vi "VI_Principal.vi"() -> ()   [LabVIEW 2024]
uses:
  <vilib>/LabVIEW Open Source Project/Epoch Date & Time/epoch.UNIX/Epoch.UNIX.lvclass
panel:
  in  "Tab Control":enum32{"Page 1", "Page 2", "Page 3"}(tab)
  out "POTENCIA  A":waveform(dbl)(graph)
  out "FASE B":waveform(dbl)
  out "POTENCIA   B":waveform(dbl)(graph)
  out "output waveform":waveform(dbl)
  out "POTENCIA CC":waveform(dbl)(graph)
  out "FASE C":dbl(graph)
  out "FASE A":waveform(dbl)(graph)
  in  "stop 2":bool
  out "Waveform Chart 3":waveform(dbl)(graph)
  in  "stop":bool
  out "Waveform Chart 2":waveform(dbl)(graph)
  out "Waveform Chart":dbl(graph)
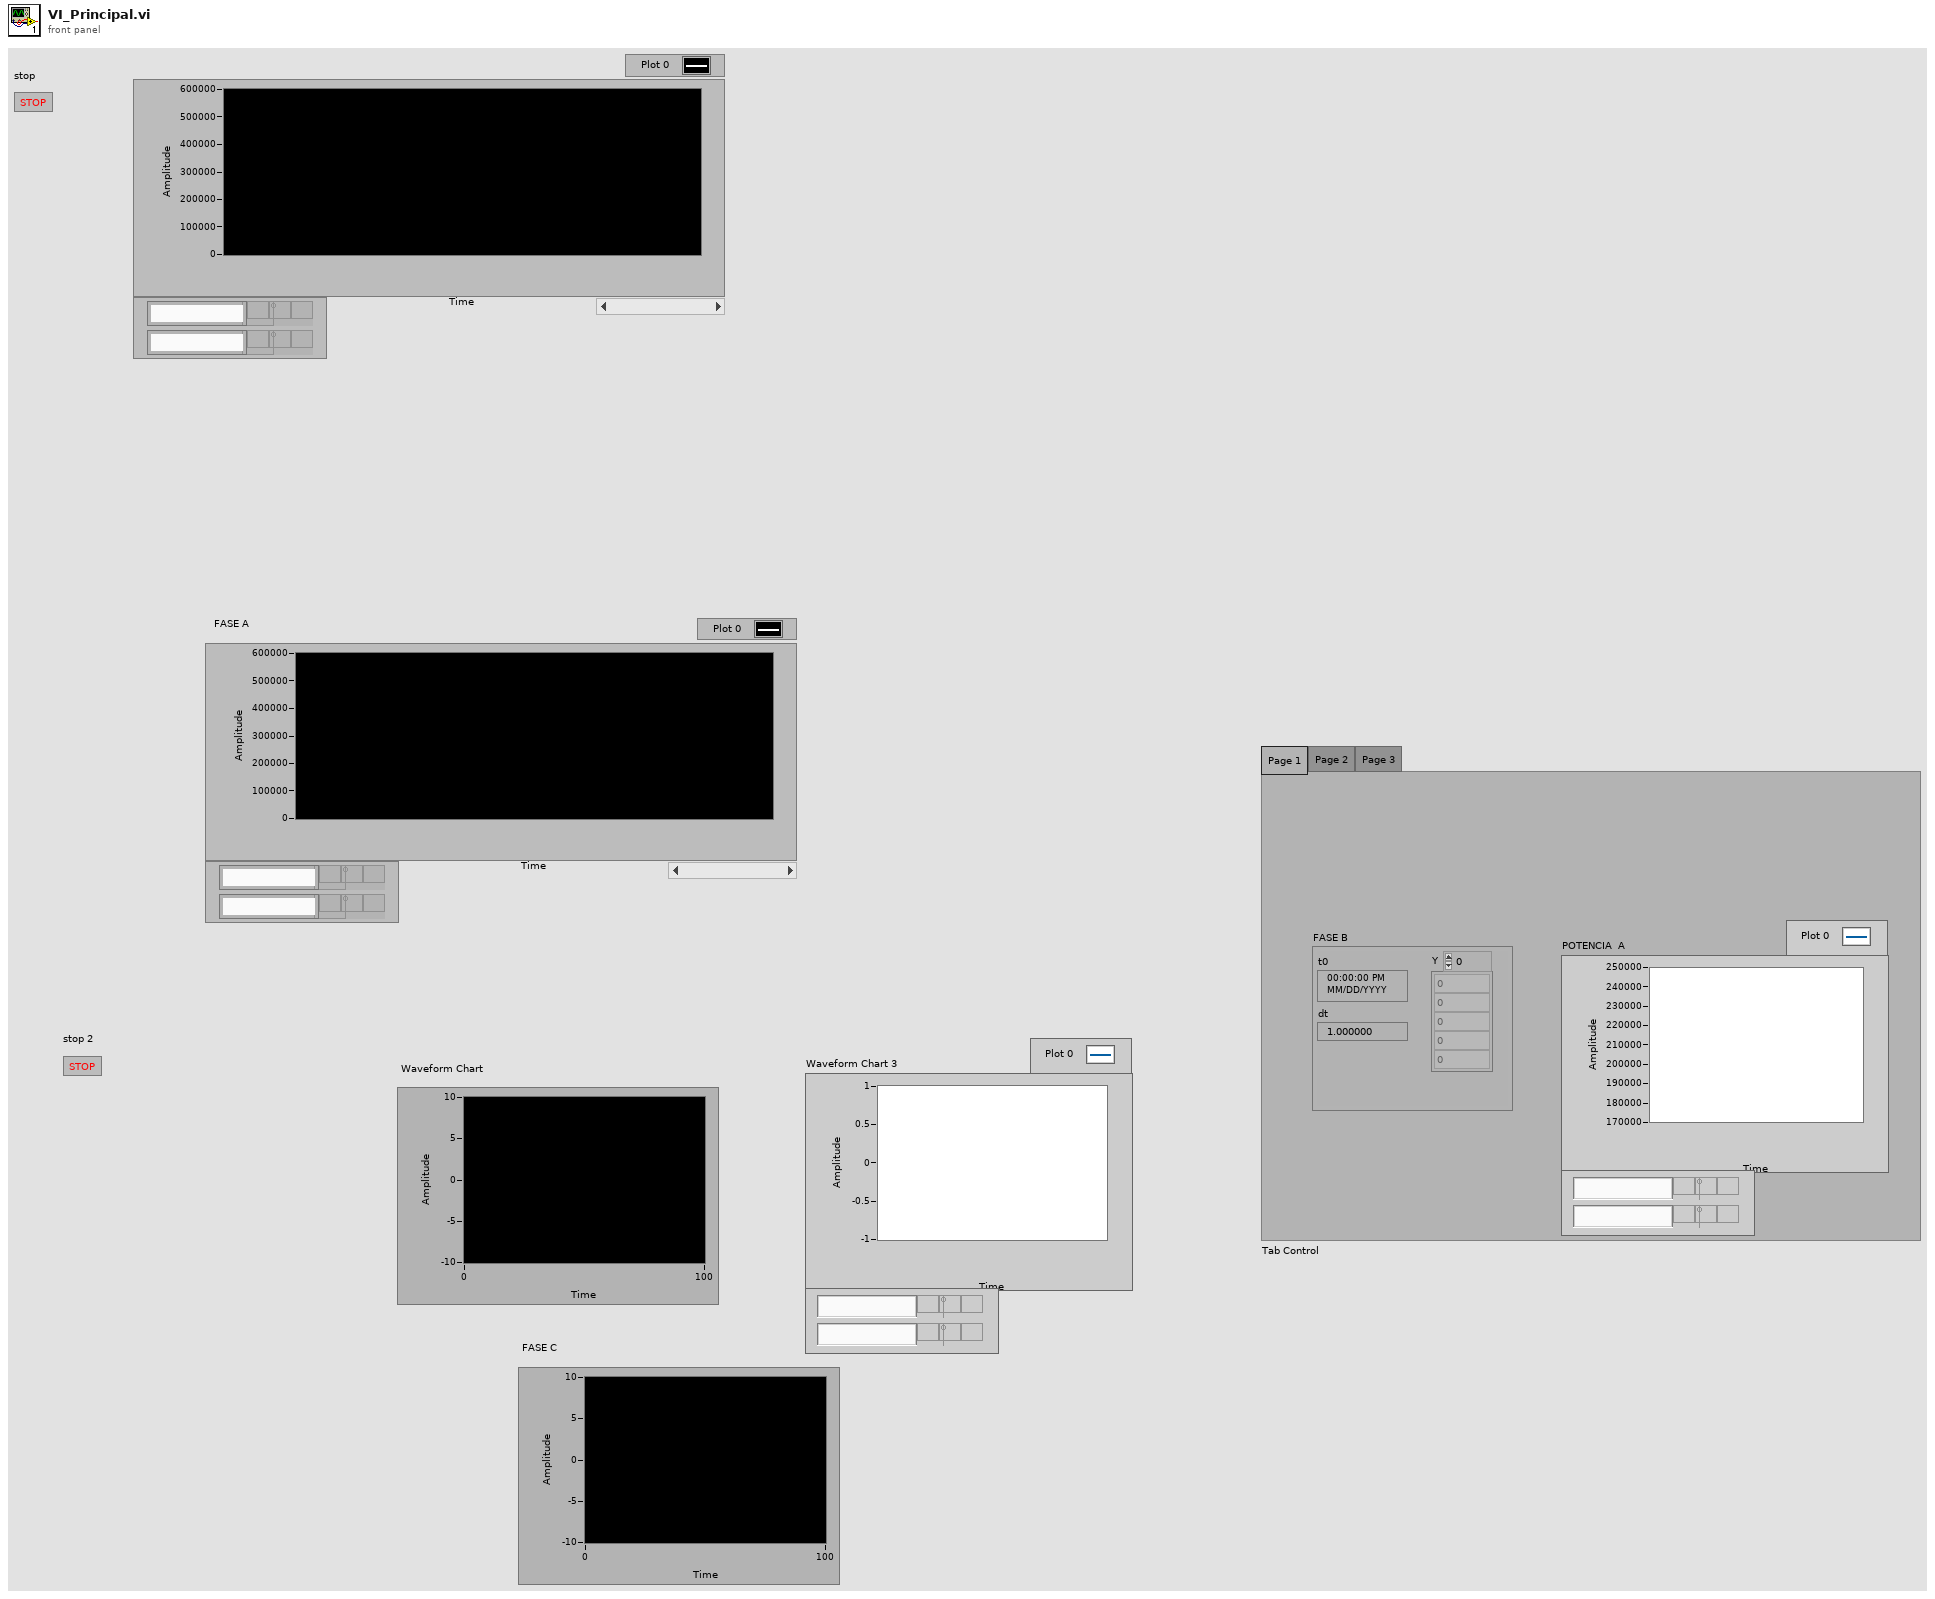
[diagram p1: front panel]
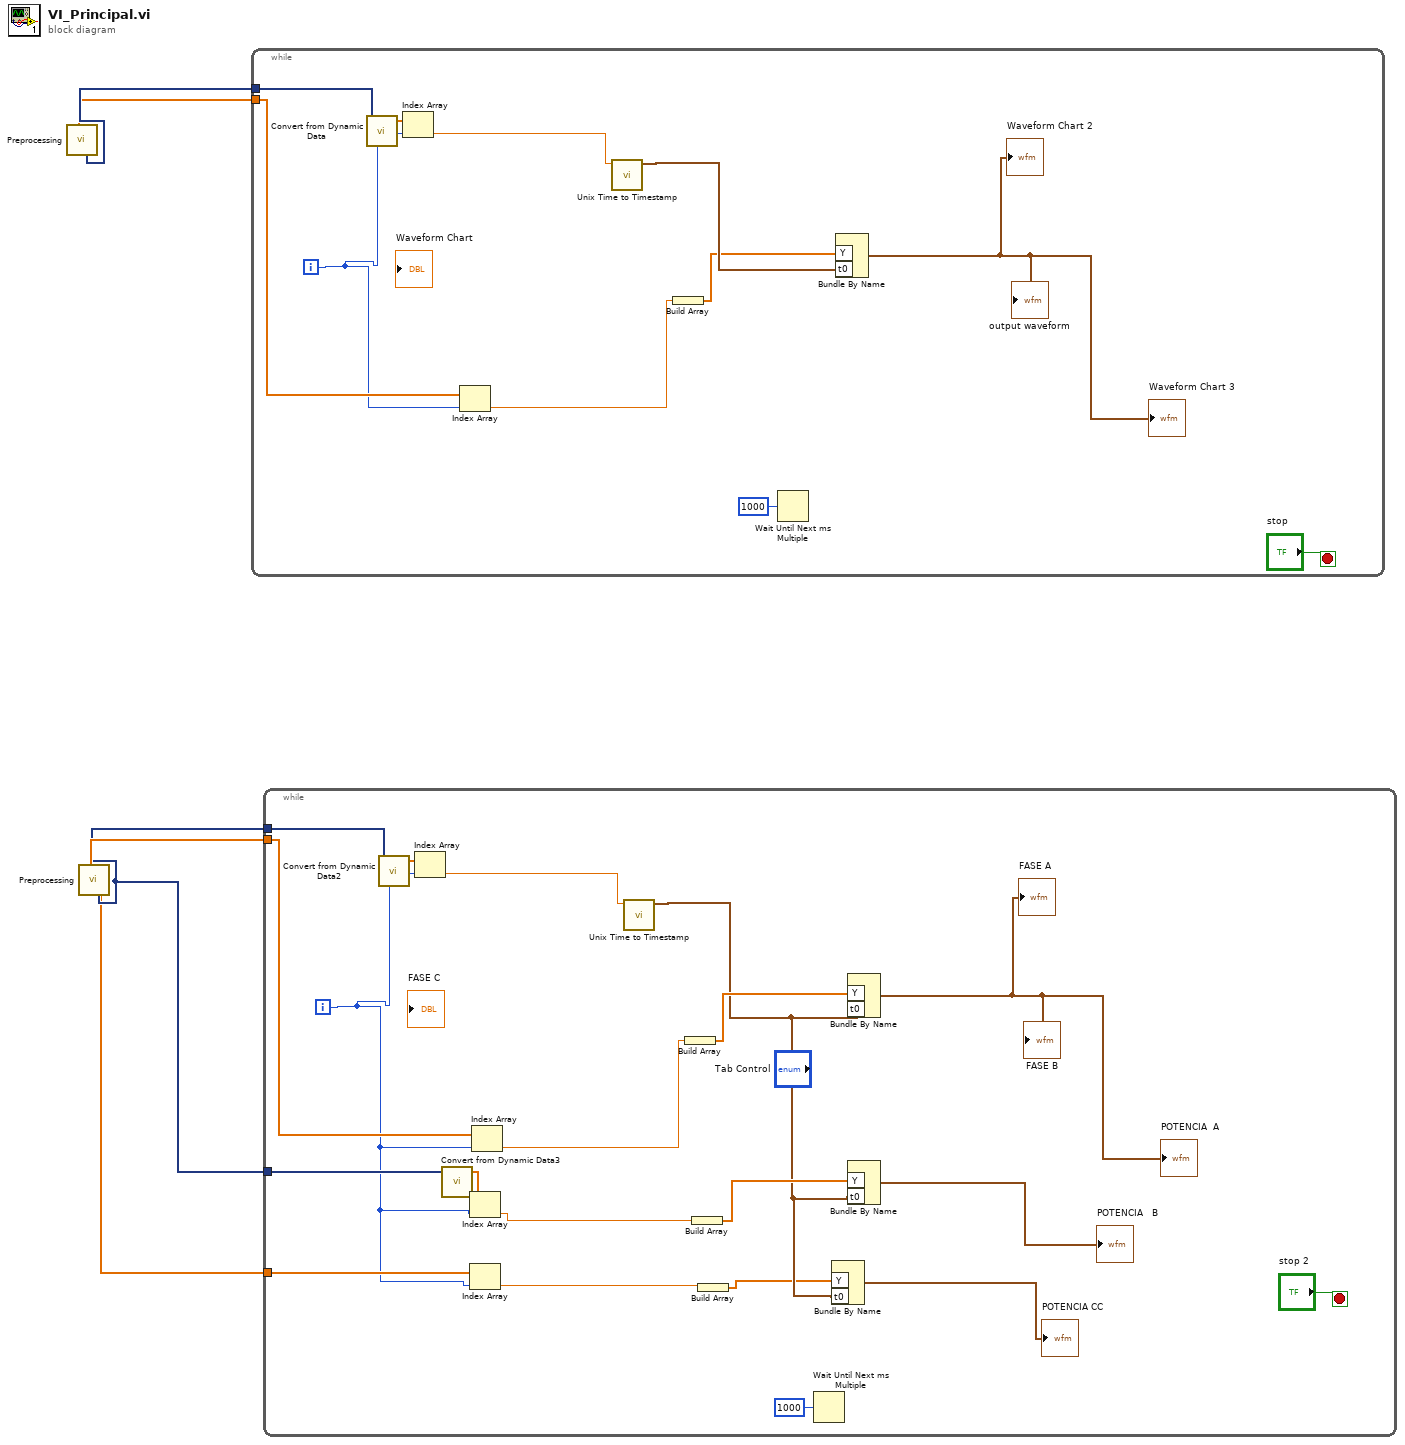
[diagram p0: block diagram]
diagram:
  n1 = call "Preprocessing.vi"() -> ("TimeStamp"=w5:dynamicdata, "Potência Ativa A"=w4:dbl[])  [unwired: 8 in, 2 out]
  n2 = call "Preprocessing.vi"() -> ("TimeStamp"=w2:dynamicdata, "Potência Ativa A 3"=w1:dbl[], "Potência Ativa A"=w3:dbl[])  [unwired: 8 in, 1 out]
  n3 = while {
    tunnel: w4 -> [w16]
    tunnel: w5 -> [w15]
    i -> [w14]
    stop <- "stop" stop-if-true
    n4 = call "Convert from Dynamic Data"("Dynamic Data Type"=w15) -> ("Array"=w6:dbl[])  [unwired: 3 in]
    n5 = Index Array(array=w6, index=w14) -> (element=w13:dbl)
    n6 = Index Array(array=w16, index=w14) -> (element=w11:dbl)
    n7 = call <vilib>:"Unix Time to Timestamp.vi"("Unix Time (s)"=w13) -> ("Timestamp"=w12:timestamp)  [unwired: 9 in, 1 out]
    n8 = Build Array(w11) -> (w10:dbl[])
    n9 = Wait Until Next ms Multiple(millisecond multiple=u32 1000) -> ()  [unwired: 1 out]
    n10 = Bundle By Name("Y"=w10, "t0"=w12) -> (→"output waveform" →"Waveform Chart 2" →"Waveform Chart 3":waveform(dbl))  [unwired: 1 in]
  }
  n11 = while {
    tunnel: w3 -> [w36]
    tunnel: w2 -> [w35]
    tunnel: w2 -> [w27]
    tunnel: w1 -> [w22]
    i -> [w21]
    stop <- "stop 2" stop-if-true
    n12 = call "Convert from Dynamic Data2"("Dynamic Data Type"=w35) -> ("Array"=w28:dbl[])  [unwired: 3 in]
    n13 = Index Array(array=w28, index=w21) -> (element=w34:dbl)
    n14 = call "Convert from Dynamic Data3"("Dynamic Data Type"=w27) -> ("Array"=w26:dbl[])  [unwired: 3 in]
    n15 = Index Array(array=w26, index=w21) -> (element=w25:dbl)
    n16 = Index Array(array=w22, index=w21) -> (element=w20:dbl)
    n17 = Index Array(array=w36, index=w21) -> (element=w33:dbl)
    n18 = call <vilib>:"Unix Time to Timestamp.vi"("Unix Time (s)"=w34) -> ("Timestamp"=w19:timestamp)  [unwired: 9 in, 1 out]
    n19 = Build Array(w33) -> (w32:dbl[])
    n20 = Build Array(w25) -> (w24:dbl[])
    n21 = Build Array(w20) -> (w18:dbl[])
    n22 = Wait Until Next ms Multiple(millisecond multiple=u32 1000) -> ()  [unwired: 1 out]
    n23 = Bundle By Name("Y"=w18, "t0"=w19) -> (→"POTENCIA CC":waveform(dbl))  [unwired: 1 in]
    n24 = Bundle By Name("Y"=w32, "t0"=w19) -> (→"FASE B" →"FASE A" →"POTENCIA  A":waveform(dbl))  [unwired: 1 in]
    n25 = Bundle By Name("Y"=w24, "t0"=w19) -> (→"POTENCIA   B":waveform(dbl))  [unwired: 1 in]
  }
